vi "十六进制U8转ASCII字符串 (子VI).vi"(11 "十六进制数值":u8 format="%xH") -> (3 "ASCII字符串输出":string)   [LabVIEW 2016, in "环境动力监测库.lvlib" / "空调库.lvlib"]
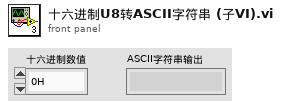
[diagram p1: front panel]
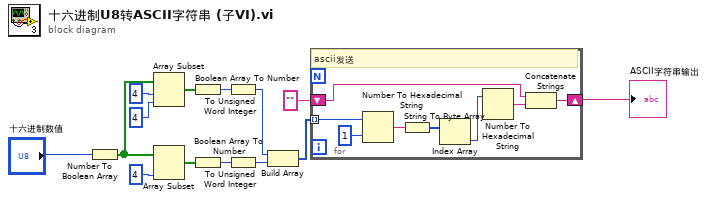
[diagram p0: block diagram]
diagram:
  n1 = Number To Boolean Array(number="十六进制数值") -> (Boolean array=w12:bool[])
  n2 = Array Subset(array=w12, index=4 ("索引"), length=4 ("长度")) -> (w9:bool[])
  n3 = Array Subset(array=w12, length=4 ("长度")) -> (w10:bool[])  [unwired: 1 in]
  n4 = Boolean Array To Number(Boolean array=w9) -> (number=w7:u32)
  n5 = Boolean Array To Number(Boolean array=w10) -> (number=w8:u32)
  n6 = To Unsigned Word Integer(number=w7) -> (unsigned 16bit integer=w5:u16)
  n7 = To Unsigned Word Integer(number=w8) -> (unsigned 16bit integer=w6:u16)
  n8 = Build Array(w5, w6) -> (w3:u16[])
  n9 = for {
    tunnel: w3 -> [w22] mode=indexing
    shift-right: [w17] -> w1
    shift-left: "" -> [w18]
    # "ascii发送"
    n10 = Number To Hexadecimal String(1:i16 1 ("宽度(-)"), 2:w22) -> (0:w16:string)
    n11 = String To Byte Array(string=w16) -> (unsigned byte array=w20:u8[])
    n12 = Index Array(array=w20) -> (element=w19:u8)  [unwired: 1 in]
    n13 = Number To Hexadecimal String(2:w19) -> (0:w15:string)  [unwired: 1 in]
    n14 = Concatenate Strings(w18, w15) -> (w17:string)
  }
  "ASCII字符串输出" <- w1
